vi "main(Test DQMH modules).vi"() -> ()   [LabVIEW 2018, in "Application.lvlib"] (continued)
        n1699 = Merge Errors(w3924, w3921) -> (w3925:errorcluster)
      }
      frame "Test Channel 9A" {
        w3967 = T9 {"command"="", "data"=variant} ("element")
        w3988 = T9 {"command"="", "data"=variant} ("element")
        w4009 = 9  # DUT channel (1-10)
        n1700 = disable-structure shown="LOGGING==TRUE" {
          disable-tunnel: w4004 -> [w4033 _]
          frame condition #0 (active) {
            n1701 = Empty String/Path?(string/path=w4033) -> (empty?=w4035:bool)
            n1702 = Select(t="Quece timeout", s=w4035, f=w4033) -> (s? t:f=w4032:string)
            n1703 = call "string log (SubVI).vi"("state Name"=w4032) -> ()  [unwired: 9 in, 2 out]
          }
          frame condition #1 {
          }
        }
        n1704 = Bundle By Name(cluster=w3988, "command"="Apps.UI Update", "data"="A") -> (w3987:T9)
        n1705 = Bundle By Name(cluster=w3988, "command"="MEAS.AllRelaysOFF2") -> (w3986:T9)
        n1706 = Bundle By Name(cluster=w3988, "command"="Apps.WaitForEvent") -> (w3985:T9)
        n1707 = Build Array(w3987, w3986, w3985) -> (w3993:T9[])
        n1708 = for {
          tunnel: [w4023] -> w3999 mode=indexing
          shift-right: [w4024] -> w4001
          shift-left: w3994 -> [w4022]
          tunnel: w3993 -> [w4021] mode=indexing
          n1709 = Unbundle By Name(w4021) -> ("command"=w4020:string, "data"=w4019:variant)
          n1710 = call "App enquece.vi"("Priority Enquece"=TRUE, "command data"=w4019, "command"=w4020, "queue in"=w4022) -> ("error out"=w4023:errorcluster, "Queue out"=w4024:refnum<queue>)  [unwired: 6 in]
        }
        n1711 = call "FGV DRV stand.vi"() -> ("Sub-Test.DCV"=w3981:bool)  [unwired: 10 in, 1 out]
        n1712 = case shown="True" w3981 {
          tunnel: [w4012 w4018] -> w4002
          frame False {
            n1713 = Build Array("WaitFor", "MEAS.requestAC") -> (w4012:string[])
          }
          frame True {
            n1714 = Build Array("Test DRV 49", "WaitForA", "MEAS.requestAC") -> (w4018:string[])
          }
        }
        n1715 = Merge Errors(w3999) -> (w3992:errorcluster)
        n1716 = Reverse 1D Array(array=w4002) -> (reversed array=w3980:string[])
        n1717 = for {
          tunnel: w3980 -> [w4030] mode=indexing
          tunnel: [w4029] -> w3998 mode=indexing
          shift-right: [w4028] -> w4000
          shift-left: w4001 -> [w4031]
          tunnel: w3992 -> [w4027]
          n1718 = call "App enquece.vi"("Priority Enquece"=TRUE, "error in (no error)"=w4027, "command"=w4030, "queue in"=w4031) -> ("error out"=w4029:errorcluster, "Queue out"=w4028:refnum<queue>)  [unwired: 6 in]
        }
        n1719 = Initialize Array(FALSE ("element"), 6 ("dimension size")) -> (w3963:bool[])
        n1720 = Initialize Array(TRUE, 1 ("dimension size")) -> (w3962:bool[])
        n1721 = Merge Errors(w3998) -> (w3997:errorcluster)
        n1722 = Replace Array Subset(array=w3963, new element=w3962) -> (w3961:bool[])  [unwired: 1 in]
        n1723 = To Variant(anything=T3."mux10_1_channel9" ("mux10_1(x6)_encode")) -> (Variant=w3978:variant)
        n1724 = To Variant(anything=T4."demux1_10_channel9" ("demux1_10(x6)_encode")) -> (Variant=w3974:variant)
        n1725 = To Variant(anything=w3961) -> (Variant=w3970:variant)
        n1726 = Bundle By Name(cluster=w3967, "command"="MEAS.mux10-1", "data"=w3978) -> (w3973:T9)
        n1727 = Bundle By Name(cluster=w3967, "command"="MEAS.demux1-10", "data"=w3974) -> (w3972:T9)
        n1728 = Bundle By Name(cluster=w3967, "command"="MEAS.eMIC", "data"=w3970) -> (w3969:T9)
        n1729 = Build Array(w3973, w3972, w3969) -> (w3996:T9[])
        n1730 = Reverse 1D Array(array=w3996) -> (reversed array=w3995:T9[])
        n1731 = for {
          tunnel: w3995 -> [w4041] mode=indexing
          tunnel: [w4038] -> w4003 mode=indexing
          tunnel: w3997 -> [w4037]
          tunnel: w4000 -> [w4042]
          n1732 = Unbundle By Name(w4041) -> ("command"=w4040:string, "data"=w4039:variant)
          n1733 = call "App enquece.vi"("Priority Enquece"=TRUE, "error in (no error)"=w4037, "command data"=w4039, "command"=w4040, "queue in"=w4042) -> ("error out"=w4038:errorcluster)  [unwired: 5 in, 1 out]
        }
        n1734 = Merge Errors(w4006, w4003) -> (w4007:errorcluster)
      }
      frame "Test Channel 10B" {
        w4049 = T9 {"command"="", "data"=variant} ("element")
        w4070 = T9 {"command"="", "data"=variant} ("element")
        w4091 = 10  # DUT channel (1-10)
        n1735 = disable-structure shown="LOGGING==TRUE" {
          disable-tunnel: w4086 -> [w4116 _]
          frame condition #0 (active) {
            n1736 = Empty String/Path?(string/path=w4116) -> (empty?=w4118:bool)
            n1737 = Select(t="Quece timeout", s=w4118, f=w4116) -> (s? t:f=w4115:string)
            n1738 = call "string log (SubVI).vi"("state Name"=w4115) -> ()  [unwired: 9 in, 2 out]
          }
          frame condition #1 {
          }
        }
        n1739 = Bundle By Name(cluster=w4070, "command"="Apps.UI Update", "data"="B") -> (w4069:T9)
        n1740 = Bundle By Name(cluster=w4070, "command"="MEAS.AllRelaysOFF2") -> (w4063:T9)
        n1741 = Bundle By Name(cluster=w4070, "command"="Apps.WaitForEvent") -> (w4068:T9)
        n1742 = Build Array(w4069, w4063, w4068) -> (w4075:T9[])
        n1743 = for {
          tunnel: [w4106] -> w4081 mode=indexing
          shift-right: [w4107] -> w4083
          shift-left: w4076 -> [w4105]
          tunnel: w4075 -> [w4104] mode=indexing
          n1744 = Unbundle By Name(w4104) -> ("command"=w4103:string, "data"=w4102:variant)
          n1745 = call "App enquece.vi"("Priority Enquece"=TRUE, "command data"=w4102, "command"=w4103, "queue in"=w4105) -> ("error out"=w4106:errorcluster, "Queue out"=w4107:refnum<queue>)  [unwired: 6 in]
        }
        n1746 = call "FGV DRV stand.vi"() -> ("Sub-Test.DCV"=w4064:bool)  [unwired: 10 in, 1 out]
        n1747 = case shown="True" w4064 {
          tunnel: [w4094 w4101] -> w4084
          frame False {
            n1748 = Build Array("WaitFor", "MEAS.requestAC") -> (w4094:string[])
          }
          frame True {
            n1749 = Build Array("Test DRV 55", "Test DRV 56", "WaitForB", "MEAS.requestAC") -> (w4101:string[])
          }
        }
        n1750 = Merge Errors(w4081) -> (w4074:errorcluster)
        n1751 = Reverse 1D Array(array=w4084) -> (reversed array=w4062:string[])
        n1752 = for {
          tunnel: w4062 -> [w4113] mode=indexing
          tunnel: [w4112] -> w4080 mode=indexing
          shift-right: [w4111] -> w4082
          shift-left: w4083 -> [w4114]
          tunnel: w4074 -> [w4110]
          n1753 = call "App enquece.vi"("Priority Enquece"=TRUE, "error in (no error)"=w4110, "command"=w4113, "queue in"=w4114) -> ("error out"=w4112:errorcluster, "Queue out"=w4111:refnum<queue>)  [unwired: 6 in]
        }
        n1754 = Merge Errors(w4080) -> (w4079:errorcluster)
        n1755 = Initialize Array(FALSE ("element"), 6 ("dimension size")) -> (w4045:bool[])
        n1756 = Initialize Array(TRUE, 2 ("dimension size")) -> (w4044:bool[])
        n1757 = Replace Array Subset(array=w4045, new element=w4044) -> (w4043:bool[])  [unwired: 1 in]
        n1758 = To Variant(anything=T3."mux10_1_channel10" ("mux10_1(x6)_encode")) -> (Variant=w4060:variant)
        n1759 = To Variant(anything=T4."demux1_10_channel10" ("demux1_10(x6)_encode")) -> (Variant=w4056:variant)
        n1760 = To Variant(anything=w4043) -> (Variant=w4052:variant)
        n1761 = Bundle By Name(cluster=w4049, "command"="MEAS.mux10-1", "data"=w4060) -> (w4055:T9)
        n1762 = Bundle By Name(cluster=w4049, "command"="MEAS.demux1-10", "data"=w4056) -> (w4054:T9)
        n1763 = Bundle By Name(cluster=w4049, "command"="MEAS.eMIC", "data"=w4052) -> (w4051:T9)
        n1764 = Build Array(w4055, w4054, w4051) -> (w4078:T9[])
        n1765 = Reverse 1D Array(array=w4078) -> (reversed array=w4077:T9[])
        n1766 = for {
          tunnel: w4077 -> [w4124] mode=indexing
          tunnel: [w4121] -> w4085 mode=indexing
          tunnel: w4079 -> [w4120]
          tunnel: w4082 -> [w4125]
          n1767 = Unbundle By Name(w4124) -> ("command"=w4123:string, "data"=w4122:variant)
          n1768 = call "App enquece.vi"("Priority Enquece"=TRUE, "error in (no error)"=w4120, "command data"=w4122, "command"=w4123, "queue in"=w4125) -> ("error out"=w4121:errorcluster)  [unwired: 5 in, 1 out]
        }
        n1769 = Merge Errors(w4088, w4085) -> (w4089:errorcluster)
      }
      frame "Test Channel 1B" {
        w4132 = T9 {"command"="", "data"=variant} ("element")
        w4153 = T9 {"command"="", "data"=variant} ("element")
        w4174 = 1  # DUT channel (1-10)
        n1770 = disable-structure shown="LOGGING==TRUE" {
          disable-tunnel: w4169 -> [w4199 _]
          frame condition #0 (active) {
            n1771 = Empty String/Path?(string/path=w4199) -> (empty?=w4201:bool)
            n1772 = Select(t="Quece timeout", s=w4201, f=w4199) -> (s? t:f=w4198:string)
            n1773 = call "string log (SubVI).vi"("state Name"=w4198) -> ()  [unwired: 9 in, 2 out]
          }
          frame condition #1 {
          }
        }
        n1774 = Bundle By Name(cluster=w4153, "command"="Apps.UI Update", "data"="B") -> (w4152:T9)
        n1775 = Bundle By Name(cluster=w4153, "command"="MEAS.AllRelaysOFF2") -> (w4146:T9)
        n1776 = Bundle By Name(cluster=w4153, "command"="Apps.WaitForEvent") -> (w4151:T9)
        n1777 = Build Array(w4152, w4146, w4151) -> (w4158:T9[])
        n1778 = for {
          tunnel: [w4189] -> w4164 mode=indexing
          shift-right: [w4190] -> w4166
          shift-left: w4159 -> [w4188]
          tunnel: w4158 -> [w4187] mode=indexing
          n1779 = Unbundle By Name(w4187) -> ("command"=w4186:string, "data"=w4185:variant)
          n1780 = call "App enquece.vi"("Priority Enquece"=TRUE, "command data"=w4185, "command"=w4186, "queue in"=w4188) -> ("error out"=w4189:errorcluster, "Queue out"=w4190:refnum<queue>)  [unwired: 6 in]
        }
        n1781 = call "FGV DRV stand.vi"() -> ("Sub-Test.DCV"=w4147:bool)  [unwired: 10 in, 1 out]
        n1782 = case shown="True" w4147 {
          tunnel: [w4177 w4184] -> w4167
          frame False {
            n1783 = Build Array("WaitFor", "MEAS.requestAC") -> (w4177:string[])
          }
          frame True {
            n1784 = Build Array("Test DRV 1", "Test DRV 2", "WaitForB", "MEAS.requestAC") -> (w4184:string[])
          }
        }
        n1785 = Merge Errors(w4164) -> (w4157:errorcluster)
        n1786 = Reverse 1D Array(array=w4167) -> (reversed array=w4145:string[])
        n1787 = for {
          tunnel: w4145 -> [w4196] mode=indexing
          tunnel: [w4195] -> w4163 mode=indexing
          shift-right: [w4194] -> w4165
          shift-left: w4166 -> [w4197]
          tunnel: w4157 -> [w4193]
          n1788 = call "App enquece.vi"("Priority Enquece"=TRUE, "error in (no error)"=w4193, "command"=w4196, "queue in"=w4197) -> ("error out"=w4195:errorcluster, "Queue out"=w4194:refnum<queue>)  [unwired: 6 in]
        }
        n1789 = Merge Errors(w4163) -> (w4162:errorcluster)
        n1790 = Initialize Array(FALSE ("element"), 6 ("dimension size")) -> (w4128:bool[])
        n1791 = Initialize Array(TRUE, 2 ("dimension size")) -> (w4127:bool[])
        n1792 = Replace Array Subset(array=w4128, new element=w4127) -> (w4126:bool[])  [unwired: 1 in]
        n1793 = To Variant(anything=T3."mux10_1_channel1" ("mux10_1(x6)_encode")) -> (Variant=w4143:variant)
        n1794 = To Variant(anything=T4."demux1_10_channel1" ("demux1_10(x6)_encode")) -> (Variant=w4139:variant)
        n1795 = To Variant(anything=w4126) -> (Variant=w4135:variant)
        n1796 = Bundle By Name(cluster=w4132, "command"="MEAS.mux10-1", "data"=w4143) -> (w4138:T9)
        n1797 = Bundle By Name(cluster=w4132, "command"="MEAS.demux1-10", "data"=w4139) -> (w4137:T9)
        n1798 = Bundle By Name(cluster=w4132, "command"="MEAS.eMIC", "data"=w4135) -> (w4134:T9)
        n1799 = Build Array(w4138, w4137, w4134) -> (w4161:T9[])
        n1800 = Reverse 1D Array(array=w4161) -> (reversed array=w4160:T9[])
        n1801 = for {
          tunnel: w4160 -> [w4207] mode=indexing
          tunnel: [w4204] -> w4168 mode=indexing
          tunnel: w4162 -> [w4203]
          tunnel: w4165 -> [w4208]
          n1802 = Unbundle By Name(w4207) -> ("command"=w4206:string, "data"=w4205:variant)
          n1803 = call "App enquece.vi"("Priority Enquece"=TRUE, "error in (no error)"=w4203, "command data"=w4205, "command"=w4206, "queue in"=w4208) -> ("error out"=w4204:errorcluster)  [unwired: 5 in, 1 out]
        }
        n1804 = Merge Errors(w4171, w4168) -> (w4172:errorcluster)
      }
      frame "Test Channel 2B" {
        w4215 = T9 {"command"="", "data"=variant} ("element")
        w4236 = T9 {"command"="", "data"=variant} ("element")
        w4257 = 2  # DUT channel (1-10)
        n1805 = disable-structure shown="LOGGING==TRUE" {
          disable-tunnel: w4252 -> [w4282 _]
          frame condition #0 (active) {
            n1806 = Empty String/Path?(string/path=w4282) -> (empty?=w4284:bool)
            n1807 = Select(t="Quece timeout", s=w4284, f=w4282) -> (s? t:f=w4281:string)
            n1808 = call "string log (SubVI).vi"("state Name"=w4281) -> ()  [unwired: 9 in, 2 out]
          }
          frame condition #1 {
          }
        }
        n1809 = Bundle By Name(cluster=w4236, "command"="Apps.UI Update", "data"="B") -> (w4235:T9)
        n1810 = Bundle By Name(cluster=w4236, "command"="MEAS.AllRelaysOFF2") -> (w4229:T9)
        n1811 = Bundle By Name(cluster=w4236, "command"="Apps.WaitForEvent") -> (w4234:T9)
        n1812 = Build Array(w4235, w4229, w4234) -> (w4241:T9[])
        n1813 = for {
          tunnel: [w4272] -> w4247 mode=indexing
          shift-right: [w4273] -> w4249
          shift-left: w4242 -> [w4271]
          tunnel: w4241 -> [w4270] mode=indexing
          n1814 = Unbundle By Name(w4270) -> ("command"=w4269:string, "data"=w4268:variant)
          n1815 = call "App enquece.vi"("Priority Enquece"=TRUE, "command data"=w4268, "command"=w4269, "queue in"=w4271) -> ("error out"=w4272:errorcluster, "Queue out"=w4273:refnum<queue>)  [unwired: 6 in]
        }
        n1816 = call "FGV DRV stand.vi"() -> ("Sub-Test.DCV"=w4230:bool)  [unwired: 10 in, 1 out]
        n1817 = case shown="True" w4230 {
          tunnel: [w4260 w4267] -> w4250
          frame False {
            n1818 = Build Array("WaitFor", "MEAS.requestAC") -> (w4260:string[])
          }
          frame True {
            n1819 = Build Array("Test DRV 7", "Test DRV 8", "WaitForB", "MEAS.requestAC") -> (w4267:string[])
          }
        }
        n1820 = Merge Errors(w4247) -> (w4240:errorcluster)
        n1821 = Reverse 1D Array(array=w4250) -> (reversed array=w4228:string[])
        n1822 = for {
          tunnel: w4228 -> [w4279] mode=indexing
          tunnel: [w4278] -> w4246 mode=indexing
          shift-right: [w4277] -> w4248
          shift-left: w4249 -> [w4280]
          tunnel: w4240 -> [w4276]
          n1823 = call "App enquece.vi"("Priority Enquece"=TRUE, "error in (no error)"=w4276, "command"=w4279, "queue in"=w4280) -> ("error out"=w4278:errorcluster, "Queue out"=w4277:refnum<queue>)  [unwired: 6 in]
        }
        n1824 = Merge Errors(w4246) -> (w4245:errorcluster)
        n1825 = Initialize Array(FALSE ("element"), 6 ("dimension size")) -> (w4211:bool[])
        n1826 = Initialize Array(TRUE, 2 ("dimension size")) -> (w4210:bool[])
        n1827 = Replace Array Subset(array=w4211, new element=w4210) -> (w4209:bool[])  [unwired: 1 in]
        n1828 = To Variant(anything=T3."mux10_1_channel2" ("mux10_1(x6)_encode")) -> (Variant=w4226:variant)
        n1829 = To Variant(anything=T4."demux1_10_channel2" ("demux1_10(x6)_encode")) -> (Variant=w4222:variant)
        n1830 = To Variant(anything=w4209) -> (Variant=w4218:variant)
        n1831 = Bundle By Name(cluster=w4215, "command"="MEAS.mux10-1", "data"=w4226) -> (w4221:T9)
        n1832 = Bundle By Name(cluster=w4215, "command"="MEAS.demux1-10", "data"=w4222) -> (w4220:T9)
        n1833 = Bundle By Name(cluster=w4215, "command"="MEAS.eMIC", "data"=w4218) -> (w4217:T9)
        n1834 = Build Array(w4221, w4220, w4217) -> (w4244:T9[])
        n1835 = Reverse 1D Array(array=w4244) -> (reversed array=w4243:T9[])
        n1836 = for {
          tunnel: w4243 -> [w4290] mode=indexing
          tunnel: [w4287] -> w4251 mode=indexing
          tunnel: w4245 -> [w4286]
          tunnel: w4248 -> [w4291]
          n1837 = Unbundle By Name(w4290) -> ("command"=w4289:string, "data"=w4288:variant)
          n1838 = call "App enquece.vi"("Priority Enquece"=TRUE, "error in (no error)"=w4286, "command data"=w4288, "command"=w4289, "queue in"=w4291) -> ("error out"=w4287:errorcluster)  [unwired: 5 in, 1 out]
        }
        n1839 = Merge Errors(w4254, w4251) -> (w4255:errorcluster)
      }
      frame "Test Channel 3B" {
        w4298 = T9 {"command"="", "data"=variant} ("element")
        w4319 = T9 {"command"="", "data"=variant} ("element")
        w4340 = 3  # DUT channel (1-10)
        n1840 = disable-structure shown="LOGGING==TRUE" {
          disable-tunnel: w4335 -> [w4365 _]
          frame condition #0 (active) {
            n1841 = Empty String/Path?(string/path=w4365) -> (empty?=w4367:bool)
            n1842 = Select(t="Quece timeout", s=w4367, f=w4365) -> (s? t:f=w4364:string)
            n1843 = call "string log (SubVI).vi"("state Name"=w4364) -> ()  [unwired: 9 in, 2 out]
          }
          frame condition #1 {
          }
        }
        n1844 = Bundle By Name(cluster=w4319, "command"="Apps.UI Update", "data"="B") -> (w4318:T9)
        n1845 = Bundle By Name(cluster=w4319, "command"="MEAS.AllRelaysOFF2") -> (w4312:T9)
        n1846 = Bundle By Name(cluster=w4319, "command"="Apps.WaitForEvent") -> (w4317:T9)
        n1847 = Build Array(w4318, w4312, w4317) -> (w4324:T9[])
        n1848 = for {
          tunnel: [w4355] -> w4330 mode=indexing
          shift-right: [w4356] -> w4332
          shift-left: w4325 -> [w4354]
          tunnel: w4324 -> [w4353] mode=indexing
          n1849 = Unbundle By Name(w4353) -> ("command"=w4352:string, "data"=w4351:variant)
          n1850 = call "App enquece.vi"("Priority Enquece"=TRUE, "command data"=w4351, "command"=w4352, "queue in"=w4354) -> ("error out"=w4355:errorcluster, "Queue out"=w4356:refnum<queue>)  [unwired: 6 in]
        }
        n1851 = call "FGV DRV stand.vi"() -> ("Sub-Test.DCV"=w4313:bool)  [unwired: 10 in, 1 out]
        n1852 = case shown="True" w4313 {
          tunnel: [w4343 w4350] -> w4333
          frame False {
            n1853 = Build Array("WaitFor", "MEAS.requestAC") -> (w4343:string[])
          }
          frame True {
            n1854 = Build Array("Test DRV 13", "Test DRV 14", "WaitForB", "MEAS.requestAC") -> (w4350:string[])
          }
        }
        n1855 = Merge Errors(w4330) -> (w4323:errorcluster)
        n1856 = Reverse 1D Array(array=w4333) -> (reversed array=w4311:string[])
        n1857 = for {
          tunnel: w4311 -> [w4362] mode=indexing
          tunnel: [w4361] -> w4329 mode=indexing
          shift-right: [w4360] -> w4331
          shift-left: w4332 -> [w4363]
          tunnel: w4323 -> [w4359]
          n1858 = call "App enquece.vi"("Priority Enquece"=TRUE, "error in (no error)"=w4359, "command"=w4362, "queue in"=w4363) -> ("error out"=w4361:errorcluster, "Queue out"=w4360:refnum<queue>)  [unwired: 6 in]
        }
        n1859 = Initialize Array(FALSE ("element"), 6 ("dimension size")) -> (w4294:bool[])
        n1860 = Merge Errors(w4329) -> (w4328:errorcluster)
        n1861 = Initialize Array(TRUE, 2 ("dimension size")) -> (w4293:bool[])
        n1862 = Replace Array Subset(array=w4294, new element=w4293) -> (w4292:bool[])  [unwired: 1 in]
        n1863 = To Variant(anything=T3."mux10_1_channel3" ("mux10_1(x6)_encode")) -> (Variant=w4309:variant)
        n1864 = To Variant(anything=T4."demux1_10_channel3" ("demux1_10(x6)_encode")) -> (Variant=w4305:variant)
        n1865 = To Variant(anything=w4292) -> (Variant=w4301:variant)
        n1866 = Bundle By Name(cluster=w4298, "command"="MEAS.mux10-1", "data"=w4309) -> (w4304:T9)
        n1867 = Bundle By Name(cluster=w4298, "command"="MEAS.demux1-10", "data"=w4305) -> (w4303:T9)
        n1868 = Bundle By Name(cluster=w4298, "command"="MEAS.eMIC", "data"=w4301) -> (w4300:T9)
        n1869 = Build Array(w4304, w4303, w4300) -> (w4327:T9[])
        n1870 = Reverse 1D Array(array=w4327) -> (reversed array=w4326:T9[])
        n1871 = for {
          tunnel: w4326 -> [w4373] mode=indexing
          tunnel: [w4370] -> w4334 mode=indexing
          tunnel: w4328 -> [w4369]
          tunnel: w4331 -> [w4374]
          n1872 = Unbundle By Name(w4373) -> ("command"=w4372:string, "data"=w4371:variant)
          n1873 = call "App enquece.vi"("Priority Enquece"=TRUE, "error in (no error)"=w4369, "command data"=w4371, "command"=w4372, "queue in"=w4374) -> ("error out"=w4370:errorcluster)  [unwired: 5 in, 1 out]
        }
        n1874 = Merge Errors(w4337, w4334) -> (w4338:errorcluster)
      }
      frame "Test Channel 4B" {
        w4381 = T9 {"command"="", "data"=variant} ("element")
        w4402 = T9 {"command"="", "data"=variant} ("element")
        w4423 = 4  # DUT channel (1-10)
        n1875 = disable-structure shown="LOGGING==TRUE" {
          disable-tunnel: w4418 -> [w4448 _]
          frame condition #0 (active) {
            n1876 = Empty String/Path?(string/path=w4448) -> (empty?=w4450:bool)
            n1877 = Select(t="Quece timeout", s=w4450, f=w4448) -> (s? t:f=w4447:string)
            n1878 = call "string log (SubVI).vi"("state Name"=w4447) -> ()  [unwired: 9 in, 2 out]
          }
          frame condition #1 {
          }
        }
        n1879 = Bundle By Name(cluster=w4402, "command"="Apps.UI Update", "data"="B") -> (w4401:T9)
        n1880 = Bundle By Name(cluster=w4402, "command"="MEAS.AllRelaysOFF2") -> (w4395:T9)
        n1881 = Bundle By Name(cluster=w4402, "command"="Apps.WaitForEvent") -> (w4400:T9)
        n1882 = Build Array(w4401, w4395, w4400) -> (w4407:T9[])
        n1883 = for {
          tunnel: [w4438] -> w4413 mode=indexing
          shift-right: [w4439] -> w4415
          shift-left: w4408 -> [w4437]
          tunnel: w4407 -> [w4436] mode=indexing
          n1884 = Unbundle By Name(w4436) -> ("command"=w4435:string, "data"=w4434:variant)
          n1885 = call "App enquece.vi"("Priority Enquece"=TRUE, "command data"=w4434, "command"=w4435, "queue in"=w4437) -> ("error out"=w4438:errorcluster, "Queue out"=w4439:refnum<queue>)  [unwired: 6 in]
        }
        n1886 = call "FGV DRV stand.vi"() -> ("Sub-Test.DCV"=w4396:bool)  [unwired: 10 in, 1 out]
        n1887 = case shown="True" w4396 {
          tunnel: [w4426 w4433] -> w4416
          frame False {
            n1888 = Build Array("WaitFor", "MEAS.requestAC") -> (w4426:string[])
          }
          frame True {
            n1889 = Build Array("Test DRV 19", "Test DRV 20", "WaitForB", "MEAS.requestAC") -> (w4433:string[])
          }
        }
        n1890 = Merge Errors(w4413) -> (w4406:errorcluster)
        n1891 = Reverse 1D Array(array=w4416) -> (reversed array=w4394:string[])
        n1892 = for {
          tunnel: w4394 -> [w4445] mode=indexing
          tunnel: [w4444] -> w4412 mode=indexing
          shift-right: [w4443] -> w4414
          shift-left: w4415 -> [w4446]
          tunnel: w4406 -> [w4442]
          n1893 = call "App enquece.vi"("Priority Enquece"=TRUE, "error in (no error)"=w4442, "command"=w4445, "queue in"=w4446) -> ("error out"=w4444:errorcluster, "Queue out"=w4443:refnum<queue>)  [unwired: 6 in]
        }
        n1894 = Initialize Array(FALSE ("element"), 6 ("dimension size")) -> (w4377:bool[])
        n1895 = Initialize Array(TRUE, 2 ("dimension size")) -> (w4376:bool[])
        n1896 = Merge Errors(w4412) -> (w4411:errorcluster)
        n1897 = Replace Array Subset(array=w4377, new element=w4376) -> (w4375:bool[])  [unwired: 1 in]
        n1898 = To Variant(anything=T3."mux10_1_channel4" ("mux10_1(x6)_encode")) -> (Variant=w4392:variant)
        n1899 = To Variant(anything=T4."demux1_10_channel4" ("demux1_10(x6)_encode")) -> (Variant=w4388:variant)
        n1900 = To Variant(anything=w4375) -> (Variant=w4384:variant)
        n1901 = Bundle By Name(cluster=w4381, "command"="MEAS.mux10-1", "data"=w4392) -> (w4387:T9)
        n1902 = Bundle By Name(cluster=w4381, "command"="MEAS.demux1-10", "data"=w4388) -> (w4386:T9)
        n1903 = Bundle By Name(cluster=w4381, "command"="MEAS.eMIC", "data"=w4384) -> (w4383:T9)
        n1904 = Build Array(w4387, w4386, w4383) -> (w4410:T9[])
        n1905 = Reverse 1D Array(array=w4410) -> (reversed array=w4409:T9[])
        n1906 = for {
          tunnel: w4409 -> [w4456] mode=indexing
          tunnel: [w4453] -> w4417 mode=indexing
          tunnel: w4411 -> [w4452]
          tunnel: w4414 -> [w4457]
          n1907 = Unbundle By Name(w4456) -> ("command"=w4455:string, "data"=w4454:variant)
          n1908 = call "App enquece.vi"("Priority Enquece"=TRUE, "error in (no error)"=w4452, "command data"=w4454, "command"=w4455, "queue in"=w4457) -> ("error out"=w4453:errorcluster)  [unwired: 5 in, 1 out]
        }
        n1909 = Merge Errors(w4420, w4417) -> (w4421:errorcluster)
      }
      frame "Test Channel 5B" {
        w4464 = T9 {"command"="", "data"=variant} ("element")
        w4485 = T9 {"command"="", "data"=variant} ("element")
        w4506 = 5  # DUT channel (1-10)
        n1910 = disable-structure shown="LOGGING==TRUE" {
          disable-tunnel: w4501 -> [w4531 _]
          frame condition #0 (active) {
            n1911 = Empty String/Path?(string/path=w4531) -> (empty?=w4533:bool)
            n1912 = Select(t="Quece timeout", s=w4533, f=w4531) -> (s? t:f=w4530:string)
            n1913 = call "string log (SubVI).vi"("state Name"=w4530) -> ()  [unwired: 9 in, 2 out]
          }
          frame condition #1 {
          }
        }
        n1914 = Bundle By Name(cluster=w4485, "command"="Apps.UI Update", "data"="B") -> (w4484:T9)
        n1915 = Bundle By Name(cluster=w4485, "command"="MEAS.AllRelaysOFF2") -> (w4478:T9)
        n1916 = Bundle By Name(cluster=w4485, "command"="Apps.WaitForEvent") -> (w4483:T9)
        n1917 = Build Array(w4484, w4478, w4483) -> (w4490:T9[])
        n1918 = for {
          tunnel: [w4521] -> w4496 mode=indexing
          shift-right: [w4522] -> w4498
          shift-left: w4491 -> [w4520]
          tunnel: w4490 -> [w4519] mode=indexing
          n1919 = Unbundle By Name(w4519) -> ("command"=w4518:string, "data"=w4517:variant)
          n1920 = call "App enquece.vi"("Priority Enquece"=TRUE, "command data"=w4517, "command"=w4518, "queue in"=w4520) -> ("error out"=w4521:errorcluster, "Queue out"=w4522:refnum<queue>)  [unwired: 6 in]
        }
        n1921 = call "FGV DRV stand.vi"() -> ("Sub-Test.DCV"=w4479:bool)  [unwired: 10 in, 1 out]
        n1922 = case shown="False" w4479 {
          tunnel: [w4509 w4516] -> w4499
          frame False {
            n1923 = Build Array("WaitFor", "MEAS.requestAC") -> (w4509:string[])
          }
          frame True {
            n1924 = Build Array("Test DRV 25", "Test DRV 26", "WaitForB", "MEAS.requestAC") -> (w4516:string[])
          }
        }
        n1925 = Merge Errors(w4496) -> (w4489:errorcluster)
        n1926 = Reverse 1D Array(array=w4499) -> (reversed array=w4477:string[])
        n1927 = for {
          tunnel: w4477 -> [w4528] mode=indexing
          tunnel: [w4527] -> w4495 mode=indexing
          shift-right: [w4526] -> w4497
          shift-left: w4498 -> [w4529]
          tunnel: w4489 -> [w4525]
          n1928 = call "App enquece.vi"("Priority Enquece"=TRUE, "error in (no error)"=w4525, "command"=w4528, "queue in"=w4529) -> ("error out"=w4527:errorcluster, "Queue out"=w4526:refnum<queue>)  [unwired: 6 in]
        }
        n1929 = Initialize Array(FALSE ("element"), 6 ("dimension size")) -> (w4460:bool[])
        n1930 = Merge Errors(w4495) -> (w4494:errorcluster)
        n1931 = Initialize Array(TRUE, 2 ("dimension size")) -> (w4459:bool[])
        n1932 = Replace Array Subset(array=w4460, new element=w4459) -> (w4458:bool[])  [unwired: 1 in]
        n1933 = To Variant(anything=T3."mux10_1_channel5" ("mux10_1(x6)_encode")) -> (Variant=w4475:variant)
        n1934 = To Variant(anything=T4."demux1_10_channel5" ("demux1_10(x6)_encode")) -> (Variant=w4471:variant)
        n1935 = To Variant(anything=w4458) -> (Variant=w4467:variant)
        n1936 = Bundle By Name(cluster=w4464, "command"="MEAS.mux10-1", "data"=w4475) -> (w4470:T9)
        n1937 = Bundle By Name(cluster=w4464, "command"="MEAS.demux1-10", "data"=w4471) -> (w4469:T9)
        n1938 = Bundle By Name(cluster=w4464, "command"="MEAS.eMIC", "data"=w4467) -> (w4466:T9)
        n1939 = Build Array(w4470, w4469, w4466) -> (w4493:T9[])
        n1940 = Reverse 1D Array(array=w4493) -> (reversed array=w4492:T9[])
        n1941 = for {
          tunnel: w4492 -> [w4539] mode=indexing
          tunnel: [w4536] -> w4500 mode=indexing
          tunnel: w4494 -> [w4535]
          tunnel: w4497 -> [w4540]
          n1942 = Unbundle By Name(w4539) -> ("command"=w4538:string, "data"=w4537:variant)
          n1943 = call "App enquece.vi"("Priority Enquece"=TRUE, "error in (no error)"=w4535, "command data"=w4537, "command"=w4538, "queue in"=w4540) -> ("error out"=w4536:errorcluster)  [unwired: 5 in, 1 out]
        }
        n1944 = Merge Errors(w4503, w4500) -> (w4504:errorcluster)
      }
      frame "Test Channel 6B" {
        w4550 = T9 {"command"="", "data"=variant} ("element")
        w4571 = 6  # DUT channel (1-10)
        n1945 = disable-structure shown="LOGGING==TRUE" {
          disable-tunnel: w4566 -> [w4632 _]
          frame condition #0 (active) {
            n1946 = Empty String/Path?(string/path=w4632) -> (empty?=w4634:bool)
            n1947 = Select(t="Quece timeout", s=w4634, f=w4632) -> (s? t:f=w4631:string)
            n1948 = call "string log (SubVI).vi"("state Name"=w4631) -> ()  [unwired: 9 in, 2 out]
          }
          frame condition #1 {
          }
        }
        n1949 = Bundle By Name(cluster=w4550, "command"="Apps.UI Update", "data"="B") -> (w4549:T9)
        n1950 = Bundle By Name(cluster=w4550, "command"="MEAS.AllRelaysOFF2") -> (w4542:T9)
        n1951 = Bundle By Name(cluster=w4550, "command"="Apps.WaitForEvent") -> (w4548:T9)
        n1952 = Build Array(w4549, w4542, w4548) -> (w4555:T9[])
        n1953 = for {
          tunnel: [w4622] -> w4561 mode=indexing
          shift-right: [w4623] -> w4563
          shift-left: w4556 -> [w4621]
          tunnel: w4555 -> [w4620] mode=indexing
          n1954 = Unbundle By Name(w4620) -> ("command"=w4619:string, "data"=w4618:variant)
          n1955 = call "App enquece.vi"("Priority Enquece"=TRUE, "command data"=w4618, "command"=w4619, "queue in"=w4621) -> ("error out"=w4622:errorcluster, "Queue out"=w4623:refnum<queue>)  [unwired: 6 in]
        }
        n1956 = Merge Errors(w4561) -> (w4554:errorcluster)
        n1957 = call "FGV DRV stand.vi"() -> ("Sub-Test.DCV"=w4544:bool)  [unwired: 10 in, 1 out]
        n1958 = case shown="True" w4544 {
          tunnel: [w4610 w4617] -> w4564
          frame False {
            n1959 = Build Array("WaitFor", "MEAS.requestAC") -> (w4610:string[])
          }
          frame True {
            n1960 = Build Array("Test DRV 31", "Test DRV 32", "WaitForB", "MEAS.requestAC") -> (w4617:string[])
          }
        }
        n1961 = Reverse 1D Array(array=w4564) -> (reversed array=w4541:string[])
        n1962 = for {
          tunnel: w4541 -> [w4629] mode=indexing
          tunnel: [w4628] -> w4560 mode=indexing
          shift-right: [w4627] -> w4562
          shift-left: w4563 -> [w4630]
          tunnel: w4554 -> [w4626]
          n1963 = call "App enquece.vi"("Priority Enquece"=TRUE, "error in (no error)"=w4626, "command"=w4629, "queue in"=w4630) -> ("error out"=w4628:errorcluster, "Queue out"=w4627:refnum<queue>)  [unwired: 6 in]
        }
        n1964 = call "FGV DRV stand.vi"() -> ("Sub-Test.DCV"=w4543:bool)  [unwired: 10 in, 1 out]
        n1965 = Merge Errors(w4560) -> (w4559:errorcluster)
        n1966 = case shown="True" w4543 {
          tunnel: [w4582 w4602] -> w4558
          frame True {
            w4580 = T9 {"command"="", "data"=variant} ("element")
            n1967 = Initialize Array(FALSE ("element"), 6 ("dimension size")) -> (w4576:bool[])
            n1968 = Initialize Array(TRUE, 2 ("dimension size")) -> (w4575:bool[])
            n1969 = Replace Array Subset(array=w4576, new element=w4575) -> (w4574:bool[])  [unwired: 1 in]
            n1970 = To Variant(anything=T3."mux10_1_channel6" ("mux10_1(x6)_encode")) -> (Variant=w4592:variant)
            n1971 = To Variant(anything=T4."demux1_10_channel6" ("demux1_10(x6)_encode")) -> (Variant=w4588:variant)
            n1972 = To Variant(anything=w4574) -> (Variant=w4584:variant)
            n1973 = Bundle By Name(cluster=w4580, "command"="MEAS.mux10-1", "data"=w4592) -> (w4587:T9)
            n1974 = Bundle By Name(cluster=w4580, "command"="MEAS.demux1-10", "data"=w4588) -> (w4586:T9)
            n1975 = Bundle By Name(cluster=w4580, "command"="MEAS.eMIC", "data"=w4584) -> (w4583:T9)
            n1976 = Build Array(w4587, w4586, w4583) -> (w4582:T9[])
          }
          frame False {
            w4600 = T9 {"command"="", "data"=variant} ("element")
            n1977 = Initialize Array(FALSE ("element"), 6 ("dimension size")) -> (w4596:bool[])
            n1978 = Initialize Array(TRUE, 2 ("dimension size")) -> (w4595:bool[])
            n1979 = Replace Array Subset(array=w4596, new element=w4595) -> (w4594:bool[])  [unwired: 1 in]
            n1980 = To Variant(anything=T4."demux1_10_channel6" ("demux1_10(x6)_encode")) -> (Variant=w4607:variant)
            n1981 = To Variant(anything=w4594) -> (Variant=w4604:variant)
            n1982 = Bundle By Name(cluster=w4600, "command"="MEAS.demux1-10", "data"=w4607) -> (w4606:T9)
            n1983 = Bundle By Name(cluster=w4600, "command"="MEAS.eMIC", "data"=w4604) -> (w4603:T9)
            n1984 = Build Array(w4606, w4603) -> (w4602:T9[])
          }
        }
        n1985 = Reverse 1D Array(array=w4558) -> (reversed array=w4557:T9[])
        n1986 = for {
          tunnel: w4557 -> [w4640] mode=indexing
          tunnel: [w4637] -> w4565 mode=indexing
          tunnel: w4559 -> [w4636]
          tunnel: w4562 -> [w4641]
          n1987 = Unbundle By Name(w4640) -> ("command"=w4639:string, "data"=w4638:variant)
          n1988 = call "App enquece.vi"("Priority Enquece"=TRUE, "error in (no error)"=w4636, "command data"=w4638, "command"=w4639, "queue in"=w4641) -> ("error out"=w4637:errorcluster)  [unwired: 5 in, 1 out]
        }
        n1989 = Merge Errors(w4568, w4565) -> (w4569:errorcluster)
      }
      frame "Test Channel 7B" {
        w4648 = T9 {"command"="", "data"=variant} ("element")
        w4669 = T9 {"command"="", "data"=variant} ("element")
        w4690 = 7  # DUT channel (1-10)
        n1990 = disable-structure shown="LOGGING==TRUE" {
          disable-tunnel: w4685 -> [w4715 _]
          frame condition #0 (active) {
            n1991 = Empty String/Path?(string/path=w4715) -> (empty?=w4717:bool)
            n1992 = Select(t="Quece timeout", s=w4717, f=w4715) -> (s? t:f=w4714:string)
            n1993 = call "string log (SubVI).vi"("state Name"=w4714) -> ()  [unwired: 9 in, 2 out]
          }
          frame condition #1 {
          }
        }
        n1994 = Bundle By Name(cluster=w4669, "command"="Apps.UI Update", "data"="B") -> (w4668:T9)
        n1995 = Bundle By Name(cluster=w4669, "command"="MEAS.AllRelaysOFF2") -> (w4662:T9)
        n1996 = Bundle By Name(cluster=w4669, "command"="Apps.WaitForEvent") -> (w4667:T9)
        n1997 = Build Array(w4668, w4662, w4667) -> (w4674:T9[])
        n1998 = for {
          tunnel: [w4705] -> w4680 mode=indexing
          shift-right: [w4706] -> w4682
          shift-left: w4675 -> [w4704]
          tunnel: w4674 -> [w4703] mode=indexing
          n1999 = Unbundle By Name(w4703) -> ("command"=w4702:string, "data"=w4701:variant)
          n2000 = call "App enquece.vi"("Priority Enquece"=TRUE, "command data"=w4701, "command"=w4702, "queue in"=w4704) -> ("error out"=w4705:errorcluster, "Queue out"=w4706:refnum<queue>)  [unwired: 6 in]
        }
        n2001 = call "FGV DRV stand.vi"() -> ("Sub-Test.DCV"=w4663:bool)  [unwired: 10 in, 1 out]
        n2002 = case shown="True" w4663 {
          tunnel: [w4693 w4700] -> w4683
          frame False {
            n2003 = Build Array("WaitFor", "MEAS.requestAC") -> (w4693:string[])
          }
          frame True {
            n2004 = Build Array("Test DRV 37", "Test DRV 38", "WaitForB", "MEAS.requestAC") -> (w4700:string[])
          }
        }
        n2005 = Merge Errors(w4680) -> (w4673:errorcluster)
        n2006 = Reverse 1D Array(array=w4683) -> (reversed array=w4661:string[])
        n2007 = for {
          tunnel: w4661 -> [w4712] mode=indexing
          tunnel: [w4711] -> w4679 mode=indexing
          shift-right: [w4710] -> w4681
          shift-left: w4682 -> [w4713]
          tunnel: w4673 -> [w4709]
          n2008 = call "App enquece.vi"("Priority Enquece"=TRUE, "error in (no error)"=w4709, "command"=w4712, "queue in"=w4713) -> ("error out"=w4711:errorcluster, "Queue out"=w4710:refnum<queue>)  [unwired: 6 in]
        }
        n2009 = Merge Errors(w4679) -> (w4678:errorcluster)
        n2010 = Initialize Array(FALSE ("element"), 6 ("dimension size")) -> (w4644:bool[])
        n2011 = Initialize Array(TRUE, 2 ("dimension size")) -> (w4643:bool[])
        n2012 = Replace Array Subset(array=w4644, new element=w4643) -> (w4642:bool[])  [unwired: 1 in]
        n2013 = To Variant(anything=T3."mux10_1_channel7" ("mux10_1(x6)_encode")) -> (Variant=w4659:variant)
        n2014 = To Variant(anything=T4."demux1_10_channel7" ("demux1_10(x6)_encode")) -> (Variant=w4655:variant)
        n2015 = To Variant(anything=w4642) -> (Variant=w4651:variant)
        n2016 = Bundle By Name(cluster=w4648, "command"="MEAS.mux10-1", "data"=w4659) -> (w4654:T9)
        n2017 = Bundle By Name(cluster=w4648, "command"="MEAS.demux1-10", "data"=w4655) -> (w4653:T9)
        n2018 = Bundle By Name(cluster=w4648, "command"="MEAS.eMIC", "data"=w4651) -> (w4650:T9)
        n2019 = Build Array(w4654, w4653, w4650) -> (w4677:T9[])
        n2020 = Reverse 1D Array(array=w4677) -> (reversed array=w4676:T9[])
        n2021 = for {
          tunnel: w4676 -> [w4723] mode=indexing
          tunnel: [w4720] -> w4684 mode=indexing
          tunnel: w4678 -> [w4719]
          tunnel: w4681 -> [w4724]
          n2022 = Unbundle By Name(w4723) -> ("command"=w4722:string, "data"=w4721:variant)
          n2023 = call "App enquece.vi"("Priority Enquece"=TRUE, "error in (no error)"=w4719, "command data"=w4721, "command"=w4722, "queue in"=w4724) -> ("error out"=w4720:errorcluster)  [unwired: 5 in, 1 out]
        }
        n2024 = Merge Errors(w4687, w4684) -> (w4688:errorcluster)
      }
      frame "Test Channel 8B" {
        w4731 = T9 {"command"="", "data"=variant} ("element")
        w4752 = T9 {"command"="", "data"=variant} ("element")
        w4773 = 8  # DUT channel (1-10)
        n2025 = disable-structure shown="LOGGING==TRUE" {
          disable-tunnel: w4768 -> [w4798 _]
          frame condition #0 (active) {
            n2026 = Empty String/Path?(string/path=w4798) -> (empty?=w4800:bool)
            n2027 = Select(t="Quece timeout", s=w4800, f=w4798) -> (s? t:f=w4797:string)
            n2028 = call "string log (SubVI).vi"("state Name"=w4797) -> ()  [unwired: 9 in, 2 out]
          }
          frame condition #1 {
          }
        }
        n2029 = Bundle By Name(cluster=w4752, "command"="Apps.UI Update", "data"="B") -> (w4751:T9)
        n2030 = Bundle By Name(cluster=w4752, "command"="MEAS.AllRelaysOFF2") -> (w4745:T9)
        n2031 = Bundle By Name(cluster=w4752, "command"="Apps.WaitForEvent") -> (w4750:T9)
        n2032 = Build Array(w4751, w4745, w4750) -> (w4757:T9[])
        n2033 = for {
          tunnel: [w4788] -> w4763 mode=indexing
          shift-right: [w4789] -> w4765
          shift-left: w4758 -> [w4787]
          tunnel: w4757 -> [w4786] mode=indexing
          n2034 = Unbundle By Name(w4786) -> ("command"=w4785:string, "data"=w4784:variant)
          n2035 = call "App enquece.vi"("Priority Enquece"=TRUE, "command data"=w4784, "command"=w4785, "queue in"=w4787) -> ("error out"=w4788:errorcluster, "Queue out"=w4789:refnum<queue>)  [unwired: 6 in]
        }
        n2036 = call "FGV DRV stand.vi"() -> ("Sub-Test.DCV"=w4746:bool)  [unwired: 10 in, 1 out]
        n2037 = case shown="True" w4746 {
          tunnel: [w4776 w4783] -> w4766
          frame False {
            n2038 = Build Array("WaitFor", "MEAS.requestAC") -> (w4776:string[])
          }
          frame True {
            n2039 = Build Array("Test DRV 43", "Test DRV 44", "WaitForB", "MEAS.requestAC") -> (w4783:string[])
          }
        }
        n2040 = Merge Errors(w4763) -> (w4756:errorcluster)
        n2041 = Reverse 1D Array(array=w4766) -> (reversed array=w4744:string[])
        n2042 = for {
          tunnel: w4744 -> [w4795] mode=indexing
          tunnel: [w4794] -> w4762 mode=indexing
          shift-right: [w4793] -> w4764
          shift-left: w4765 -> [w4796]
          tunnel: w4756 -> [w4792]
          n2043 = call "App enquece.vi"("Priority Enquece"=TRUE, "error in (no error)"=w4792, "command"=w4795, "queue in"=w4796) -> ("error out"=w4794:errorcluster, "Queue out"=w4793:refnum<queue>)  [unwired: 6 in]
        }
        n2044 = Initialize Array(FALSE ("element"), 6 ("dimension size")) -> (w4727:bool[])
        n2045 = Initialize Array(TRUE, 2 ("dimension size")) -> (w4726:bool[])
        n2046 = Merge Errors(w4762) -> (w4761:errorcluster)
        n2047 = Replace Array Subset(array=w4727, new element=w4726) -> (w4725:bool[])  [unwired: 1 in]
        n2048 = To Variant(anything=T3."mux10_1_channel8" ("mux10_1(x6)_encode")) -> (Variant=w4742:variant)
        n2049 = To Variant(anything=T4."demux1_10_channel8" ("demux1_10(x6)_encode")) -> (Variant=w4738:variant)
        n2050 = To Variant(anything=w4725) -> (Variant=w4734:variant)
        n2051 = Bundle By Name(cluster=w4731, "command"="MEAS.mux10-1", "data"=w4742) -> (w4737:T9)
        n2052 = Bundle By Name(cluster=w4731, "command"="MEAS.demux1-10", "data"=w4738) -> (w4736:T9)
        n2053 = Bundle By Name(cluster=w4731, "command"="MEAS.eMIC", "data"=w4734) -> (w4733:T9)
        n2054 = Build Array(w4737, w4736, w4733) -> (w4760:T9[])
        n2055 = Reverse 1D Array(array=w4760) -> (reversed array=w4759:T9[])
        n2056 = for {
          tunnel: w4759 -> [w4806] mode=indexing
          tunnel: [w4803] -> w4767 mode=indexing
          tunnel: w4761 -> [w4802]
          tunnel: w4764 -> [w4807]
          n2057 = Unbundle By Name(w4806) -> ("command"=w4805:string, "data"=w4804:variant)
          n2058 = call "App enquece.vi"("Priority Enquece"=TRUE, "error in (no error)"=w4802, "command data"=w4804, "command"=w4805, "queue in"=w4807) -> ("error out"=w4803:errorcluster)  [unwired: 5 in, 1 out]
        }
        n2059 = Merge Errors(w4770, w4767) -> (w4771:errorcluster)
      }
      frame "Test Channel 9B" {
        w4814 = T9 {"command"="", "data"=variant} ("element")
        w4835 = T9 {"command"="", "data"=variant} ("element")
        w4856 = 9  # DUT channel (1-10)
        n2060 = disable-structure shown="LOGGING==TRUE" {
          disable-tunnel: w4851 -> [w4881 _]
          frame condition #0 (active) {
            n2061 = Empty String/Path?(string/path=w4881) -> (empty?=w4883:bool)
            n2062 = Select(t="Quece timeout", s=w4883, f=w4881) -> (s? t:f=w4880:string)
            n2063 = call "string log (SubVI).vi"("state Name"=w4880) -> ()  [unwired: 9 in, 2 out]
          }
          frame condition #1 {
          }
        }
        n2064 = Bundle By Name(cluster=w4835, "command"="Apps.UI Update", "data"="B") -> (w4834:T9)
        n2065 = Bundle By Name(cluster=w4835, "command"="MEAS.AllRelaysOFF2") -> (w4828:T9)
        n2066 = Bundle By Name(cluster=w4835, "command"="Apps.WaitForEvent") -> (w4833:T9)
        n2067 = Build Array(w4834, w4828, w4833) -> (w4840:T9[])
        n2068 = for {
          tunnel: [w4871] -> w4846 mode=indexing
          shift-right: [w4872] -> w4848
          shift-left: w4841 -> [w4870]
          tunnel: w4840 -> [w4869] mode=indexing
          n2069 = Unbundle By Name(w4869) -> ("command"=w4868:string, "data"=w4867:variant)
          n2070 = call "App enquece.vi"("Priority Enquece"=TRUE, "command data"=w4867, "command"=w4868, "queue in"=w4870) -> ("error out"=w4871:errorcluster, "Queue out"=w4872:refnum<queue>)  [unwired: 6 in]
        }
        n2071 = call "FGV DRV stand.vi"() -> ("Sub-Test.DCV"=w4829:bool)  [unwired: 10 in, 1 out]
        n2072 = case shown="False" w4829 {
          tunnel: [w4859 w4866] -> w4849
          frame False {
            n2073 = Build Array("WaitFor", "MEAS.requestAC") -> (w4859:string[])
          }
          frame True {
            n2074 = Build Array("Test DRV 49", "Test DRV 50", "WaitForB", "MEAS.requestAC") -> (w4866:string[])
          }
        }
        n2075 = Merge Errors(w4846) -> (w4839:errorcluster)
        n2076 = Reverse 1D Array(array=w4849) -> (reversed array=w4827:string[])
        n2077 = for {
          tunnel: w4827 -> [w4878] mode=indexing
          tunnel: [w4877] -> w4845 mode=indexing
          shift-right: [w4876] -> w4847
          shift-left: w4848 -> [w4879]
          tunnel: w4839 -> [w4875]
          n2078 = call "App enquece.vi"("Priority Enquece"=TRUE, "error in (no error)"=w4875, "command"=w4878, "queue in"=w4879) -> ("error out"=w4877:errorcluster, "Queue out"=w4876:refnum<queue>)  [unwired: 6 in]
        }
        n2079 = Initialize Array(FALSE ("element"), 6 ("dimension size")) -> (w4810:bool[])
        n2080 = Initialize Array(TRUE, 2 ("dimension size")) -> (w4809:bool[])
        n2081 = Replace Array Subset(array=w4810, new element=w4809) -> (w4808:bool[])  [unwired: 1 in]
        n2082 = Merge Errors(w4845) -> (w4844:errorcluster)
        n2083 = To Variant(anything=T3."mux10_1_channel9" ("mux10_1(x6)_encode")) -> (Variant=w4825:variant)
        n2084 = To Variant(anything=T4."demux1_10_channel9" ("demux1_10(x6)_encode")) -> (Variant=w4821:variant)
        n2085 = To Variant(anything=w4808) -> (Variant=w4817:variant)
        n2086 = Bundle By Name(cluster=w4814, "command"="MEAS.mux10-1", "data"=w4825) -> (w4820:T9)
        n2087 = Bundle By Name(cluster=w4814, "command"="MEAS.demux1-10", "data"=w4821) -> (w4819:T9)
        n2088 = Bundle By Name(cluster=w4814, "command"="MEAS.eMIC", "data"=w4817) -> (w4816:T9)
        n2089 = Build Array(w4820, w4819, w4816) -> (w4843:T9[])
        n2090 = Reverse 1D Array(array=w4843) -> (reversed array=w4842:T9[])
        n2091 = for {
          tunnel: w4842 -> [w4889] mode=indexing
          tunnel: [w4886] -> w4850 mode=indexing
          tunnel: w4844 -> [w4885]
          tunnel: w4847 -> [w4890]
          n2092 = Unbundle By Name(w4889) -> ("command"=w4888:string, "data"=w4887:variant)
          n2093 = call "App enquece.vi"("Priority Enquece"=TRUE, "error in (no error)"=w4885, "command data"=w4887, "command"=w4888, "queue in"=w4890) -> ("error out"=w4886:errorcluster)  [unwired: 5 in, 1 out]
        }
        n2094 = Merge Errors(w4853, w4850) -> (w4854:errorcluster)
      }
      frame "Test Channel 10C" {
        w4897 = T9 {"command"="", "data"=variant} ("element")
        w4918 = T9 {"command"="", "data"=variant} ("element")
        w4939 = 10  # DUT channel (1-10)
        n2095 = disable-structure shown="LOGGING==TRUE" {
          disable-tunnel: w4934 -> [w4965 _]
          frame condition #0 (active) {
            n2096 = Empty String/Path?(string/path=w4965) -> (empty?=w4967:bool)
            n2097 = Select(t="Quece timeout", s=w4967, f=w4965) -> (s? t:f=w4964:string)
            n2098 = call "string log (SubVI).vi"("state Name"=w4964) -> ()  [unwired: 9 in, 2 out]
          }
          frame condition #1 {
          }
        }
        n2099 = Bundle By Name(cluster=w4918, "command"="Apps.UI Update", "data"="C") -> (w4917:T9)
        n2100 = Bundle By Name(cluster=w4918, "command"="MEAS.AllRelaysOFF2") -> (w4916:T9)
        n2101 = Bundle By Name(cluster=w4918, "command"="Apps.WaitForEvent") -> (w4915:T9)
        n2102 = Build Array(w4917, w4916, w4915) -> (w4923:T9[])
        n2103 = for {
          tunnel: [w4955] -> w4929 mode=indexing
          shift-right: [w4956] -> w4931
          shift-left: w4924 -> [w4954]
          tunnel: w4923 -> [w4953] mode=indexing
          n2104 = Unbundle By Name(w4953) -> ("command"=w4952:string, "data"=w4951:variant)
          n2105 = call "App enquece.vi"("Priority Enquece"=TRUE, "command data"=w4951, "command"=w4952, "queue in"=w4954) -> ("error out"=w4955:errorcluster, "Queue out"=w4956:refnum<queue>)  [unwired: 6 in]
        }
        n2106 = call "FGV DRV stand.vi"() -> ("Sub-Test.DCV"=w4912:bool)  [unwired: 10 in, 1 out]
        n2107 = case shown="True" w4912 {
          tunnel: [w4942 w4950] -> w4932
          frame False {
            n2108 = Build Array("WaitFor", "MEAS.requestAC") -> (w4942:string[])
          }
          frame True {
            n2109 = Build Array("Test DRV 55", "Test DRV 56", "Test DRV 57", "WaitForC", "MEAS.requestAC") -> (w4950:string[])
          }
        }
        n2110 = Merge Errors(w4929) -> (w4922:errorcluster)
        n2111 = Reverse 1D Array(array=w4932) -> (reversed array=w4911:string[])
        n2112 = for {
          tunnel: w4911 -> [w4962] mode=indexing
          tunnel: [w4961] -> w4928 mode=indexing
          shift-right: [w4960] -> w4930
          shift-left: w4931 -> [w4963]
          tunnel: w4922 -> [w4959]
          n2113 = call "App enquece.vi"("Priority Enquece"=TRUE, "error in (no error)"=w4959, "command"=w4962, "queue in"=w4963) -> ("error out"=w4961:errorcluster, "Queue out"=w4960:refnum<queue>)  [unwired: 6 in]
        }
        n2114 = Initialize Array(FALSE ("element"), 6 ("dimension size")) -> (w4893:bool[])
        n2115 = Merge Errors(w4928) -> (w4927:errorcluster)
        n2116 = Initialize Array(TRUE, 3 ("dimension size")) -> (w4892:bool[])
        n2117 = Replace Array Subset(array=w4893, new element=w4892) -> (w4891:bool[])  [unwired: 1 in]
        n2118 = To Variant(anything=T3."mux10_1_channel10" ("mux10_1(x6)_encode")) -> (Variant=w4908:variant)
        n2119 = To Variant(anything=T4."demux1_10_channel10" ("demux1_10(x6)_encode")) -> (Variant=w4904:variant)
        n2120 = To Variant(anything=w4891) -> (Variant=w4900:variant)
        n2121 = Bundle By Name(cluster=w4897, "command"="MEAS.mux10-1", "data"=w4908) -> (w4903:T9)
        n2122 = Bundle By Name(cluster=w4897, "command"="MEAS.demux1-10", "data"=w4904) -> (w4902:T9)
        n2123 = Bundle By Name(cluster=w4897, "command"="MEAS.eMIC", "data"=w4900) -> (w4899:T9)
        n2124 = Build Array(w4903, w4902, w4899) -> (w4926:T9[])
        n2125 = Reverse 1D Array(array=w4926) -> (reversed array=w4925:T9[])
        n2126 = for {
          tunnel: w4925 -> [w4973] mode=indexing
          tunnel: [w4970] -> w4933 mode=indexing
          tunnel: w4927 -> [w4969]
          tunnel: w4930 -> [w4974]
          n2127 = Unbundle By Name(w4973) -> ("command"=w4972:string, "data"=w4971:variant)
          n2128 = call "App enquece.vi"("Priority Enquece"=TRUE, "error in (no error)"=w4969, "command data"=w4971, "command"=w4972, "queue in"=w4974) -> ("error out"=w4970:errorcluster)  [unwired: 5 in, 1 out]
        }
        n2129 = Merge Errors(w4936, w4933) -> (w4937:errorcluster)
      }
      frame "Test Channel 1C" {
        w4981 = T9 {"command"="", "data"=variant} ("element")
        w5002 = T9 {"command"="", "data"=variant} ("element")
        w5023 = 1  # DUT channel (1-10)
        n2130 = disable-structure shown="LOGGING==TRUE" {
          disable-tunnel: w5018 -> [w5049 _]
          frame condition #0 (active) {
            n2131 = Empty String/Path?(string/path=w5049) -> (empty?=w5051:bool)
            n2132 = Select(t="Quece timeout", s=w5051, f=w5049) -> (s? t:f=w5048:string)
            n2133 = call "string log (SubVI).vi"("state Name"=w5048) -> ()  [unwired: 9 in, 2 out]
          }
          frame condition #1 {
          }
        }
        n2134 = Bundle By Name(cluster=w5002, "command"="Apps.UI Update", "data"="C") -> (w5001:T9)
        n2135 = Bundle By Name(cluster=w5002, "command"="MEAS.AllRelaysOFF2") -> (w5000:T9)
        n2136 = Bundle By Name(cluster=w5002, "command"="Apps.WaitForEvent") -> (w4999:T9)
